vi "find_file_type.vi"(9 "字符串":string, 11 "簇 2":T1) -> (1 "路径":path, 2 "是否是文件":bool, 3 "结果字符串":string)   [LabVIEW 2018, in "UI.lvlib"]
uses:
  UI.lvlib
  <vilib>/Utility/xml.llb/Read From XML File(string).vi
  <vilib>/regexp/Match Regular Expression.xnode
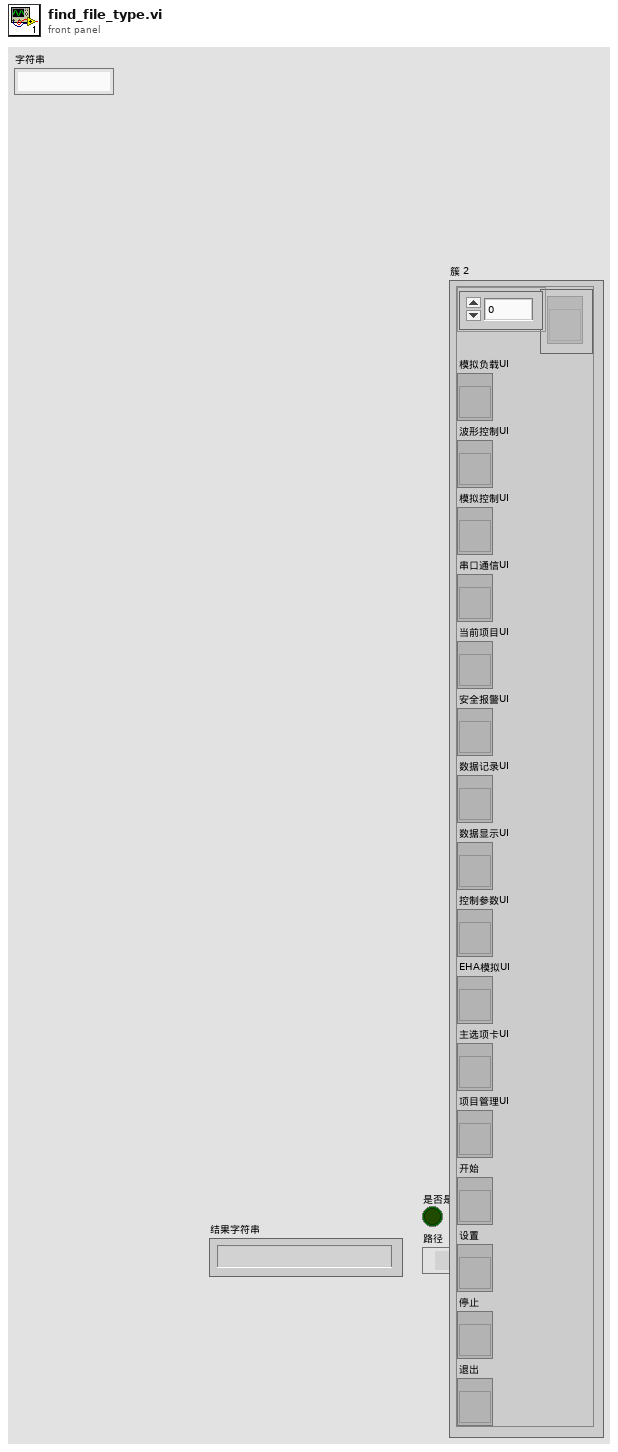
[diagram p1: front panel]
types:
  T1 = typedef "引用簇.ctl" = cluster{"数组":refnum<vi>[], "模拟负载UI":refnum<vi>, "波形控制UI":refnum<vi>, "模拟控制UI":refnum<vi>, "串口通信UI":refnum<vi>, "当前项目UI":refnum<vi>, "安全报警UI":refnum<vi>, "数据记录UI":refnum<vi>, "数据显示UI":refnum<vi>, "控制参数UI":refnum<vi>, "EHA模拟UI":refnum<vi>, "主选项卡UI":refnum<vi>, "项目管理UI":refnum<vi>, "开始":refnum<vi>, "设置":refnum<vi>, "停止":refnum<vi>, "退出":refnum<vi>}
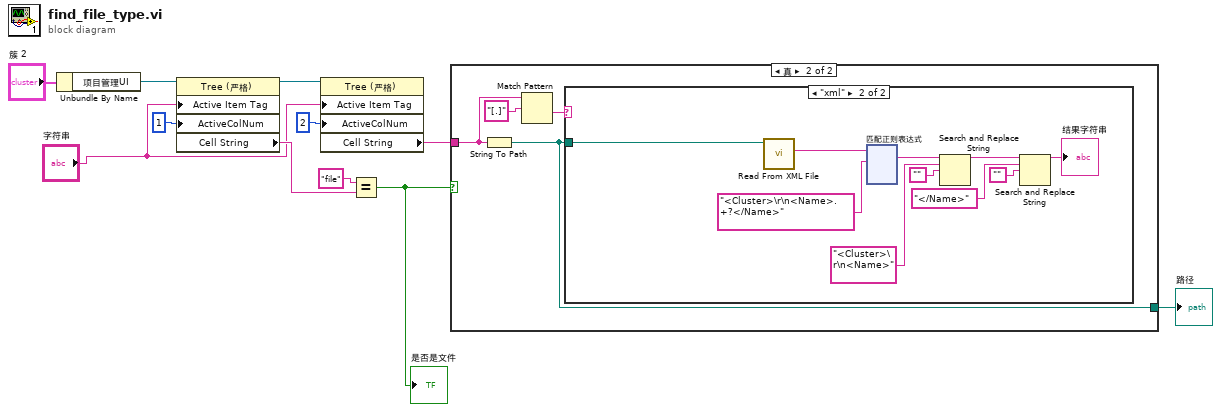
[diagram p0: block diagram]
diagram:
  n1 = Unbundle By Name("簇 2") -> ("项目管理UI"=w4:refnum<vi>)
  n2 = property class="Tree (严格)"(reference=w4, "Active Item Tag"="字符串", "ActiveColNum"=1 ("活动单元格:活动列数")) -> (reference out=w7:refnum<vi>, "Cell String"=w9:string)  [unwired: 1 in, 1 out]
  n3 = property class="Tree (严格)"(reference=w7, "Active Item Tag"="字符串", "ActiveColNum"=2 ("活动单元格:活动列数")) -> ("Cell String"=w8:string)  [unwired: 1 in, 2 out]
  n4 = Equal?(x="file", y=w9) -> (x = y?=w11:bool)
  "是否是文件" <- w11
  n5 = case shown="真" w11 {
    tunnel: w8 -> [_ w13]
    tunnel: [_ w12] -> w3
    frame False {
    }
    frame True {
      n6 = String To Path(string=w13) -> (path=w12:path)
      n7 = Match Pattern(string=w13, regular expression="[.]" ("正则表达式")) -> (after substring=w14:string)  [unwired: 1 in, 3 out]
      n8 = case shown="\"xml\"" w14 {
        tunnel: w12 -> [_ w25]
        frame Default {
        }
        frame "xml" {
          n9 = call-poly <vilib>:"Read From XML File.vi"("XML File Path"=w25) -> ("XML Elements"=w24:string)  [unwired: 8 in, 2 out]
          n10 = xnode "匹配正则表达式"("输入字符串"=w24, "正则表达式"="<Cluster>\r\n<Name>.+?</Name>") -> ("所有匹配"=w22:string)  [unwired: 4 in, 4 out]
          n11 = Search and Replace String(input string=w22, search string="<Cluster>\r\n<Name>" ("搜索字符串"), replace string="") -> (result string=w19:string)  [unwired: 5 in, 3 out]
          n12 = Search and Replace String(input string=w19, search string="</Name>" ("搜索字符串"), replace string="" ("替换字符串(\"\")")) -> (result string=→"结果字符串":string)  [unwired: 5 in, 3 out]
        }
      }
    }
  }
  "路径" <- w3
